vi "HexWordCheck2.vi"(10 "array":u8[](array[numeric]), 11 "Input Array":u8[](array[numeric])) -> (3 "Boolean":bool)   [LabVIEW 2012]
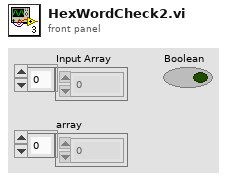
[diagram p1: front panel]
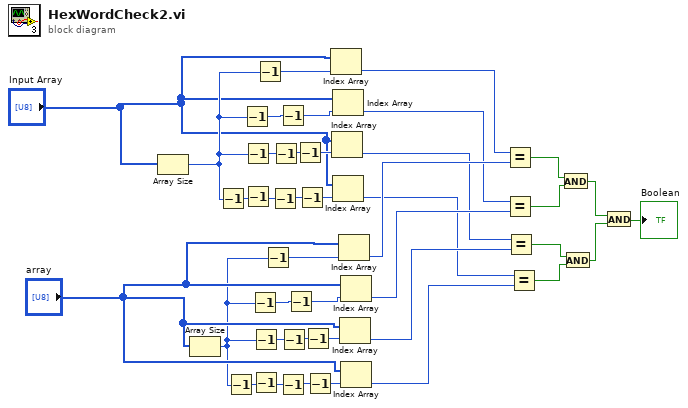
[diagram p0: block diagram]
diagram:
  n1 = Array Size(array="Input Array") -> (size(s)=w11:i32)
  n2 = Array Size(array="array") -> (size(s)=w22:i32)
  n3 = Decrement(x=w11) -> (x-1=w10:i32)
  n4 = Decrement(x=w22) -> (x-1=w21:i32)
  n5 = Decrement(x=w11) -> (x-1=w9:i32)
  n6 = Decrement(x=w11) -> (x-1=w16:i32)
  n7 = Decrement(x=w10) -> (x-1=w13:i32)
  n8 = Decrement(x=w22) -> (x-1=w20:i32)
  n9 = Decrement(x=w22) -> (x-1=w32:i32)
  n10 = Decrement(x=w21) -> (x-1=w29:i32)
  n11 = Decrement(x=w11) -> (x-1=w12:i32)
  n12 = Decrement(x=w22) -> (x-1=w23:i32)
  n13 = Decrement(x=w13) -> (x-1=w14:i32)
  n14 = Decrement(x=w16) -> (x-1=w6:i32)
  n15 = Decrement(x=w9) -> (x-1=w8:i32)
  n16 = Decrement(x=w29) -> (x-1=w30:i32)
  n17 = Decrement(x=w32) -> (x-1=w17:i32)
  n18 = Decrement(x=w20) -> (x-1=w19:i32)
  n19 = Decrement(x=w6) -> (x-1=w7:i32)
  n20 = Decrement(x=w14) -> (x-1=w15:i32)
  n21 = Decrement(x=w17) -> (x-1=w18:i32)
  n22 = Decrement(x=w30) -> (x-1=w31:i32)
  n23 = Index Array(array="Input Array", index=w12) -> (element=w4:u8)
  n24 = Index Array(array="Input Array", index=w7) -> (element=w2:u8)
  n25 = Index Array(array="Input Array", index=w8) -> (element=w3:u8)
  n26 = Index Array(array="Input Array", index=w15) -> (element=w1:u8)
  n27 = Index Array(array="array", index=w23) -> (element=w28:u8)
  n28 = Index Array(array="array", index=w18) -> (element=w26:u8)
  n29 = Index Array(array="array", index=w19) -> (element=w27:u8)
  n30 = Index Array(array="array", index=w31) -> (element=w25:u8)
  n31 = Equal?(x=w4, y=w28) -> (x = y?=w33:bool)
  n32 = Equal?(x=w3, y=w27) -> (x = y?=w37:bool)
  n33 = Equal?(x=w2, y=w26) -> (x = y?=w36:bool)
  n34 = Equal?(x=w1, y=w25) -> (x = y?=w35:bool)
  n35 = And(x=w33, y=w37) -> (x .and. y?=w38:bool)
  n36 = And(x=w36, y=w35) -> (x .and. y?=w39:bool)
  n37 = And(x=w38, y=w39) -> (x .and. y?=→"Boolean":bool)
